vi "Blinking BAP4B.vi"(8 "mode set":T3, 10 "system state in":T1) -> (2 "system state out":T1)   [LabVIEW 2014]
doc: "Blinking BAP4B\n\nSets the lights for the Blinking State according to the mode. Transitions between \"blink on\" and \"blink off\" and updates the system state based off of time remaining and change state.\n\nBeverly Abadines\nPHY 350\nP4"
uses:
  typedefs/control mode enum.ctl
  typedefs/system state cluster.ctl
  typedefs/state enum.ctl
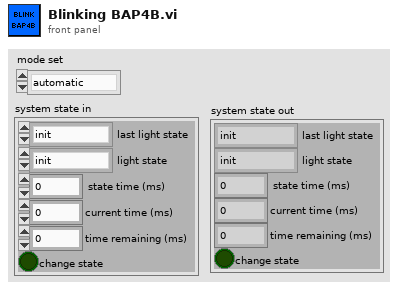
[diagram p1: front panel]
types:
  T1 = typedef "system state cluster.ctl" = cluster{"last light state":T2, "light state":T2, "state time (ms)":i32, "current time (ms)":i32, "time remaining (ms)":i32, "change state":bool}
  T2 = typedef "state enum.ctl" = enum16{"init", "idle", "left turn E", "go EW", "caution EW", "left turn W", "left turn N", "go NS", "caution NS", "left turn S", "blink on", "blink off", "all on test", "exit"}
  T3 = typedef "control mode enum.ctl" = enum16{"automatic", "blinking", "all on test"}
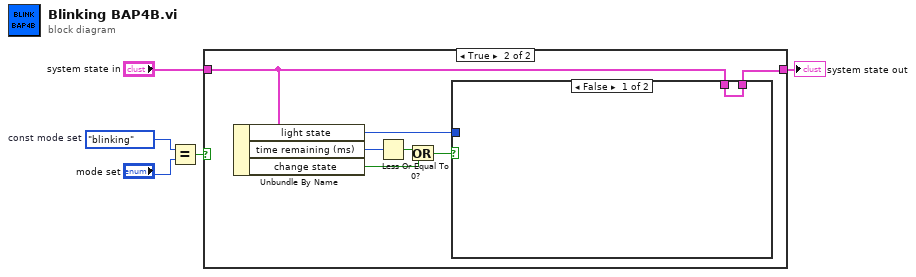
[diagram p0: block diagram]
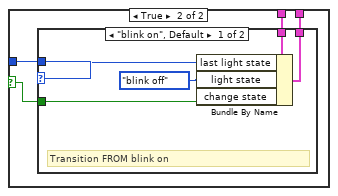
[diagram p3: hidden frame]
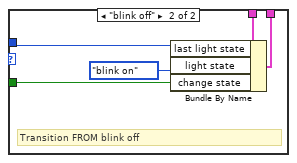
[diagram p4: hidden frame]
diagram:
  w1 = control_mode_enum."blinking"  # const mode set
  n1 = Equal?(x=w1, y="mode set") -> (x = y?=w4:bool)
  n2 = case shown="True" w4 {
    tunnel: "system state in" -> [w6 w12]
    tunnel: [w6 w13] -> w3
    frame False {
    }
    frame True {
      n3 = Unbundle By Name(w12) -> ("light state"=w11:T2, "time remaining (ms)"=w10:i32, "change state"=w7:bool)
      n4 = Less Or Equal To 0?(x=w10) -> (x <= 0?=w8:bool)
      n5 = Or(x=w8, y=w7) -> (x .or. y?=w9:bool)
      n6 = case shown="False" w9 {
        selector: w9 -> [_ w16]
        tunnel: [w14 w18] -> w13
        tunnel: w12 -> [w14 w17]
        tunnel: w11 -> [_ w15]
        frame False {
        }
        frame True {
          n7 = case shown="\"blink on\", Default" w15 {
            tunnel: w17 -> [w22 w28]
            tunnel: [w21 w26] -> w18
            tunnel: w15 -> [w20 w25]
            tunnel: w16 -> [w19 w24]
            frame "blink on", Default {
              # "Transition FROM blink on"
              n8 = Bundle By Name(cluster=w22, "last light state"=w20, "light state"=state_enum."blink off" ("const light state"), "change state"=w19) -> (w21:T1)
            }
            frame "blink off" {
              # "Transition FROM blink off"
              n9 = Bundle By Name(cluster=w28, "last light state"=w25, "light state"=state_enum."blink on" ("const light state"), "change state"=w24) -> (w26:T1)
            }
          }
        }
      }
    }
  }
  "system state out" <- w3
